vi "Self-Test.vi"(8 "error in (no error)":errorcluster, 11 "VISA resource name":refnum<visa-resource-name>) -> (0 "error out":errorcluster, 1 "Self-Test Result Message":string, 2 "Self-Test Result Code":string, 3 "VISA resource name out":refnum<visa-resource-name>)   [LabVIEW 2017, in "Sefram DAS220.lvlib"]
doc: "Runs the instrument's self-test routine and returns the test results."
uses:
  <instrlib>/Sefram DAS220/Sefram DAS220.lvlib
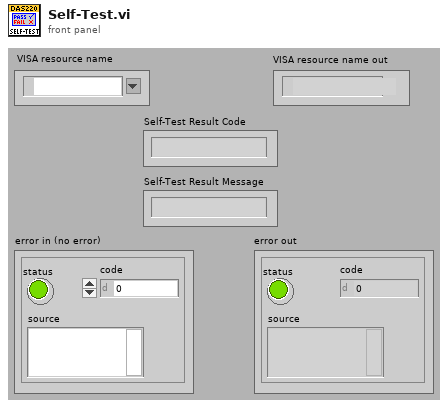
[diagram p1: front panel]
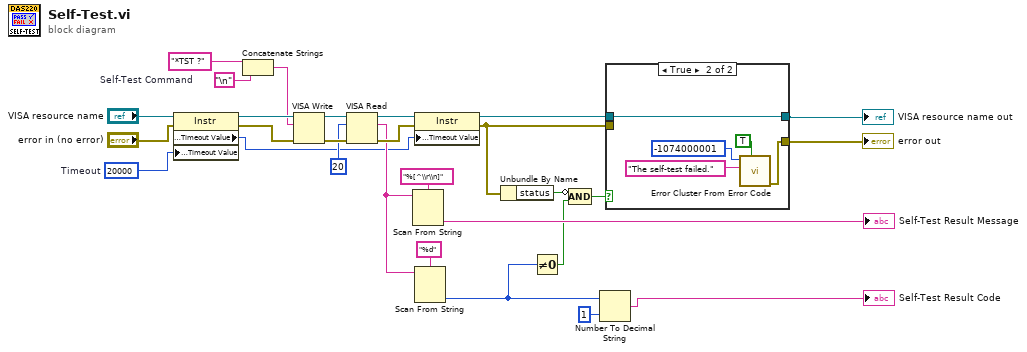
[diagram p0: block diagram]
diagram:
  w17 = u32 20000  # Timeout
  w8 = "*TST ?"  # Self-Test Command
  n1 = property class="Instr"(reference="VISA resource name", error in="error in (no error)", "General Settings:Timeout Value"=w17) -> (reference out=w15:refnum<visa-resource-name>, error out=w16:errorcluster, "General Settings:Timeout Value"=w14:u32)
  n2 = Concatenate Strings(w8, "\n") -> (w6:string)
  n3 = VISA Write(VISA resource name=w15, write buffer=w6, error in (no error)=w16) -> (VISA resource name out=w24:refnum<visa-resource-name>, error out=w23:errorcluster)  [unwired: 1 out]
  n4 = VISA Read(VISA resource name=w24, byte count=u32 20 ("byte count (20)"), error in (no error)=w23) -> (VISA resource name out=w26:refnum<visa-resource-name>, read buffer=w19:string, error out=w25:errorcluster)  [unwired: 1 out]
  n5 = Scan From String(format string="%[^\\r\\n]" ("Format String"), input string=w19) -> (output 1=→"Self-Test Result Message":string)  [unwired: 3 in, 3 out]
  n6 = property class="Instr"(reference=w26, error in=w25, "General Settings:Timeout Value"=w14) -> (reference out=w13:refnum<visa-resource-name>, error out=w12:errorcluster)
  n7 = Scan From String(format string="%d", input string=w19) -> (output 1=w3:i32)  [unwired: 3 in, 3 out]
  n8 = Unbundle By Name(w12) -> ("status"=w10:bool)
  n9 = Not Equal To 0?(x=w3) -> (x != 0?=w11:bool)
  n10 = Compound Arithmetic op=AND(invert w10, w11) -> (w9:bool)
  n11 = Number To Decimal String(number=w3, width (-)=i16 1) -> (decimal integer string=→"Self-Test Result Code":string)
  n12 = case shown="True" w9 {
    tunnel: w13 -> [w30 w35]
    tunnel: w12 -> [w29 _]
    tunnel: [w29 w31] -> w4
    tunnel: [w30 w35] -> w5
    frame False {
    }
    frame True {
      n13 = call <vilib>:"Error Cluster From Error Code.vi"("show call chain? (False)"=TRUE, "error message (\"\")"="The self-test failed." ("Source (VI Name)"), "error code (0)"=-1074000001 ("Code")) -> ("error out"=w31:errorcluster)  [unwired: 6 in]
    }
  }
  "VISA resource name out" <- w5
  "error out" <- w4
